vi "NewWeightFile.vi"(8 "error in (no error)":errorcluster, 10 "RC No":string, 11 "connection reference":T1) -> (0 "error out":errorcluster, 2 "Array":string[][](array[string]), 3 "connection reference out":T1)   [LabVIEW 2012]
uses:
  <vilib>/addons/database/Connection.llb/Conn ObjectReference.ctl
  <vilib>/addons/database/_DB Variant To Data/Database Variant To Data.xnode
  <vilib>/addons/database/NI_Database_API.lvlib
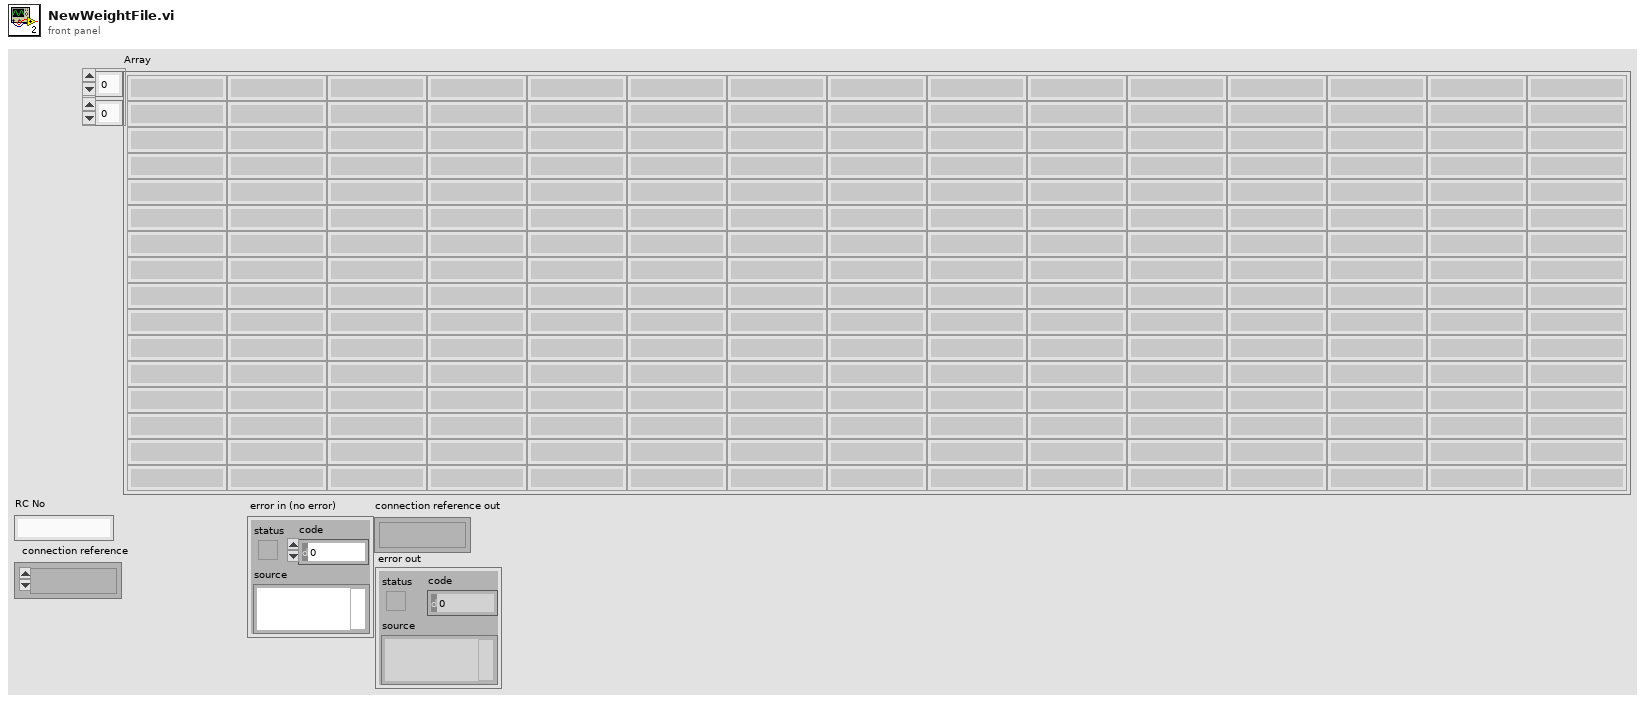
[diagram p1: front panel]
types:
  T1 = typedef "NI_Database_API.lvlib/Conn ObjectReference.ctl" = refnum<k1>
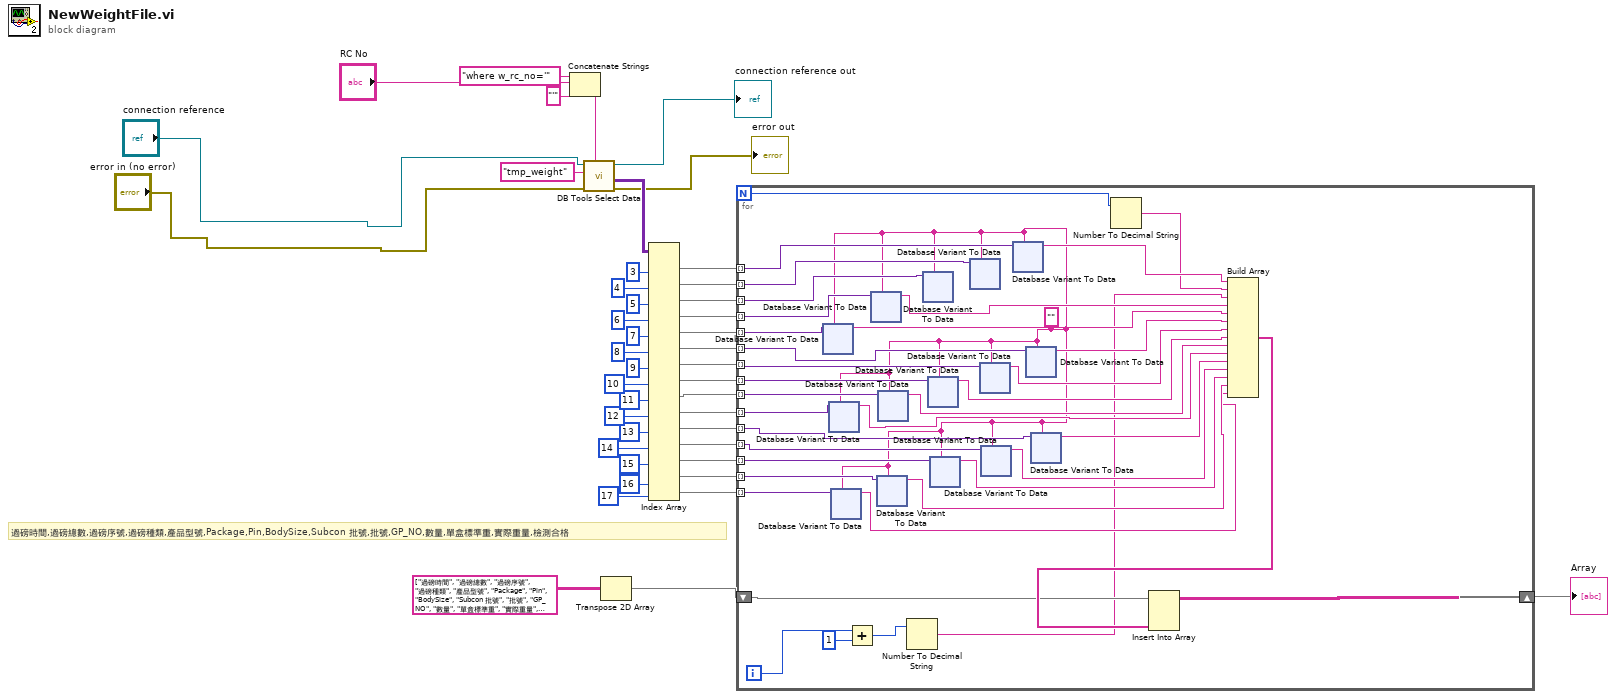
[diagram p0: block diagram]
diagram:
  # "過磅時間,過磅總數,過磅序號,過磅種類,產品型號,Package,Pin,BodySize,Subcon 批號,批號,GP_NO,數量,單盒標準重,實際重量,檢測合格"
  n1 = Concatenate Strings("where w_rc_no='" ("string"), "RC No", "'" ("string")) -> (w6:string)
  n2 = call <vilib>:"DB Tools Select Data.vi"("condition"=w6, "error in (no error)"="error in (no error)", "table"="tmp_weight", "connection reference"="connection reference") -> ("error out"=→"error out":errorcluster, "data"=w42:variant[][], "connection reference out"=→"connection reference out":T1)  [unwired: 2 in]
  n3 = Transpose 2D Array(2D array=string[][] [["過磅時間"], ["過磅總數"], ["過磅序號"], ["過磅種類"], ["產品型號"], ["Package"], ["Pin"], ["BodySize"], ["Subcon 批號"], ["批號"], ["GP_NO"], ["數量"], ["單盒標準重"], ["實際重量"], ["檢測合格"]] ("array")) -> (transposed array=w9:string[][])
  n4 = Index Array(array=w42, index (col) #1=3 ("disabled index (col)"), index (col) #2=4 ("index (col)"), index (col) #3=5 ("index (col)"), index (col) #4=6 ("index (col)"), index (col) #5=7 ("index (col)"), index (col) #6=8 ("index (col)"), index (col) #7=9 ("index (col)"), index (col) #8=10 ("index (col)"), index (col) #9=11 ("index (col)"), index (col) #10=12 ("index (col)"), index (col) #11=13 ("index (col)"), index (col) #12=14 ("index (col)"), index (col) #13=15 ("index (col)"), index (col) #14=16 ("index (col)"), index (col) #15=17 ("index (col)")) -> (element #1=w27:variant[], element #2=w26:variant[], element #3=w25:variant[], element #4=w24:variant[], element #5=w23:variant[], element #6=w22:variant[], element #7=w21:variant[], element #8=w20:variant[], element #9=w19:variant[], element #10=w18:variant[], element #11=w17:variant[], element #12=w16:variant[], element #13=w15:variant[], element #14=w14:variant[], element #15=w12:variant[])  [unwired: 15 in]
  n5 = for {
    N -> [w49]
    tunnel: w27 -> [w81] mode=indexing
    tunnel: w26 -> [w80] mode=indexing
    tunnel: w25 -> [w79] mode=indexing
    tunnel: w24 -> [w78] mode=indexing
    tunnel: w23 -> [w77] mode=indexing
    tunnel: w22 -> [w76] mode=indexing
    tunnel: w21 -> [w75] mode=indexing
    tunnel: w20 -> [w74] mode=indexing
    tunnel: w19 -> [w73] mode=indexing
    tunnel: w18 -> [w72] mode=indexing
    tunnel: w17 -> [w71] mode=indexing
    tunnel: w16 -> [w70] mode=indexing
    tunnel: w15 -> [w69] mode=indexing
    tunnel: w14 -> [w68] mode=indexing
    shift-right: [w54] -> w11
    shift-left: w9 -> [w53]
    tunnel: w12 -> [w52] mode=indexing
    i -> [w47]
    w51 = ""
    n6 = xnode "Database Variant To Data"("database variant"=w77, "type"=w51) -> ("data"=w65:string)  [unwired: 1 in, 1 out]
    n7 = xnode "Database Variant To Data"("database variant"=w72, "type"=w51) -> ("data"=w60:string)  [unwired: 1 in, 1 out]
    n8 = xnode "Database Variant To Data"("database variant"=w52, "type"=w51) -> ("data"=w50:string)  [unwired: 1 in, 1 out]
    n9 = Add(x=w47, y=1) -> (x+y=w45:i32)
    n10 = xnode "Database Variant To Data"("database variant"=w78, "type"=w51) -> ("data"=w66:string)  [unwired: 1 in, 1 out]
    n11 = xnode "Database Variant To Data"("database variant"=w68, "type"=w51) -> ("data"=w56:string)  [unwired: 1 in, 1 out]
    n12 = xnode "Database Variant To Data"("database variant"=w73, "type"=w51) -> ("data"=w61:string)  [unwired: 1 in, 1 out]
    n13 = Number To Decimal String(number=w45) -> (decimal integer string=w44:string)  [unwired: 1 in]
    n14 = xnode "Database Variant To Data"("database variant"=w79, "type"=w51) -> ()  [unwired: 1 in, 2 out]
    n15 = xnode "Database Variant To Data"("database variant"=w74, "type"=w51) -> ("data"=w62:string)  [unwired: 1 in, 1 out]
    n16 = xnode "Database Variant To Data"("database variant"=w69, "type"=w51) -> ("data"=w57:string)  [unwired: 1 in, 1 out]
    n17 = xnode "Database Variant To Data"("database variant"=w80, "type"=w51) -> ()  [unwired: 1 in, 2 out]
    n18 = xnode "Database Variant To Data"("database variant"=w75, "type"=w51) -> ("data"=w63:string)  [unwired: 1 in, 1 out]
    n19 = xnode "Database Variant To Data"("database variant"=w70, "type"=w51) -> ("data"=w58:string)  [unwired: 1 in, 1 out]
    n20 = xnode "Database Variant To Data"("database variant"=w81, "type"=w51) -> ("data"=w67:string)  [unwired: 1 in, 1 out]
    n21 = xnode "Database Variant To Data"("database variant"=w76, "type"=w51) -> ("data"=w64:string)  [unwired: 1 in, 1 out]
    n22 = xnode "Database Variant To Data"("database variant"=w71, "type"=w51) -> ("data"=w59:string)  [unwired: 1 in, 1 out]
    n23 = Number To Decimal String(number=w49) -> (decimal integer string=w48:string)  [unwired: 1 in]
    n24 = Build Array(w67, w48, w44, w66, w65, w64, w63, w62, w61, w60, w59, w58, w57, w56, w50) -> (w55:string[])
    n25 = Insert Into Array(array=w53, new element=w55) -> (w54:string[][])  [unwired: 2 in]
  }
  "Array" <- w11
